vi "subMatchedFilter.vi"(0 "Symbol Stream":cdb[][](array[numeric]), 5 "pulse shaping filter coefficients":dbl[](array[numeric]) caption="Matched FIlter coefficients" format="%.2f", 9 "samples per symbol (16)":i32=16, 11 "error in (no error)":errorcluster) -> (4 "Transmit Packets":cdb[][](array[numeric]), 15 "error out":errorcluster)   [LabVIEW 2011]
uses:
  <vilib>/addons/Modulation/Analog/controls/Complex Data Waveform.ctl
  <vilib>/addons/Modulation/Digital/General/MT Apply Matched Filter (Generic).vi
  <vilib>/addons/Modulation/niDMT.lvlib
  <vilib>/addons/Modulation/niAMT.lvlib
panel:
  in  "symbol rate (Hz)":dbl=1.0
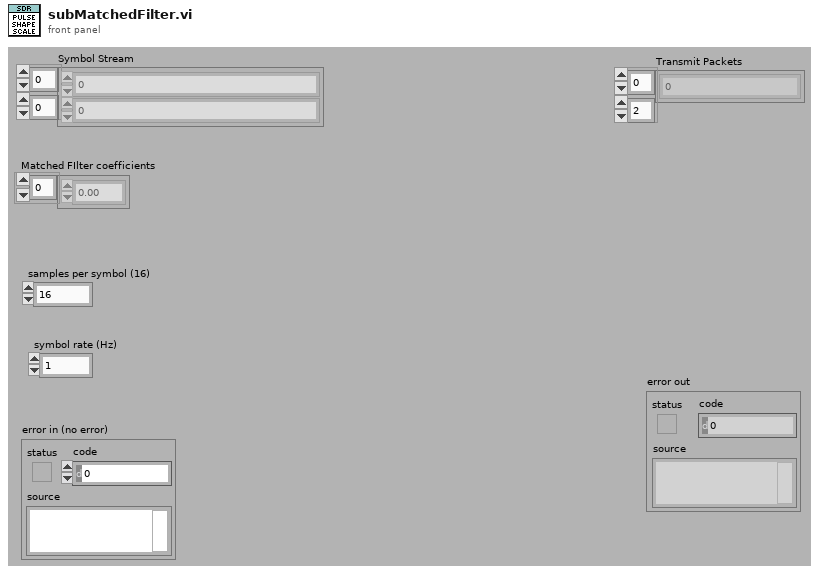
[diagram p1: front panel]
types:
  T1 = typedef "niAMT.lvlib/Complex Data Waveform.ctl" = cluster{"t0":dbl, "dt":dbl, "Y":cdb[]}
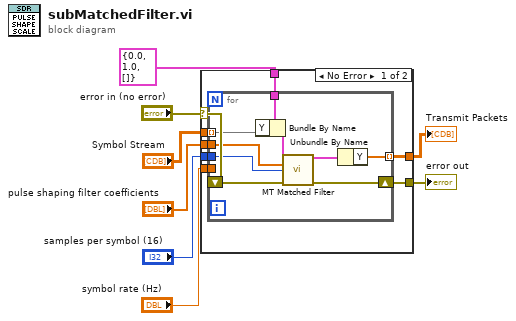
[diagram p0: block diagram]
diagram:
  n1 = case shown="No Error" "error in (no error)" {
    selector: "error in (no error)" -> [w10 w26]
    tunnel: [w14 w26] -> w7
    tunnel: "Symbol Stream" -> [w15 _]
    tunnel: "samples per symbol (16)" -> [w11 _]
    tunnel: [w16 _] -> w3
    tunnel: "pulse shaping filter coefficients" -> [w13 _]
    tunnel: "symbol rate (Hz)" -> [w12 _]
    tunnel: T1 {"t0"=0.0, "dt"=1.0, "Y"=[]} ("input complex waveform") -> [w9 _]
    frame No Error {
      n2 = for {
        tunnel: w15 -> [w19] mode=indexing
        shift-right: [w23] -> w14
        shift-left: w10 -> [w24]
        tunnel: [w25] -> w16 mode=indexing
        tunnel: w13 -> [w22]
        tunnel: w12 -> [_]
        tunnel: w11 -> [w21]
        tunnel: w9 -> [w20]
        n3 = Bundle By Name(cluster=w20, "Y"=w19) -> (w18:T1)
        n4 = call-poly <vilib>:"MT Matched Filter.vi"("input complex waveform"=w18, "matched filter coefficients"=w22, "samples per symbol (16)"=w21, "error in (no error)"=w24) -> ("output complex waveform"=w17:T1, "error out"=w23:errorcluster)  [unwired: 10 in]
        n5 = Unbundle By Name(w17) -> ("Y"=w25:cdb[])
      }
    }
    frame Error {
    }
  }
  "error out" <- w7
  "Transmit Packets" <- w3
